vi "cm_State Change.vi"(2 "Action 2":T1 caption="Action") -> (6 "Action":T1)   [LabVIEW 2012, in "Channel Monitor.xctl"]
doc: "Changes the State Changed? flag to TRUE"
uses:
  Channel Monitor.xctl
  <vilib>/_xctls/Action.ctl
  <vilib>/_xctls/XControlSupport.lvlib
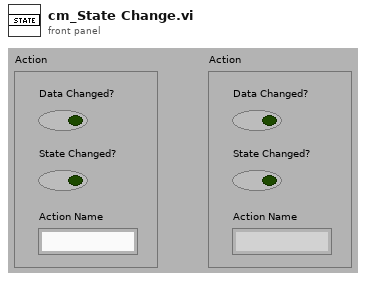
[diagram p1: front panel]
types:
  T1 = typedef "XControlSupport.lvlib/Action.ctl" = cluster{"Data Changed?":bool, "State Changed?":bool, "Action Name":string}
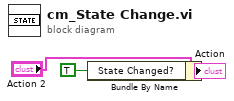
[diagram p0: block diagram]
diagram:
  n1 = Bundle By Name(cluster="Action 2", "State Changed?"=TRUE) -> (→"Action":T1)
